vi "Digitizer Analyze_DCOffset.vi"(7 "Pins":string[](array[string])=["Xout"], 8 "error in (no error)":errorcluster, 9 "Published Data Id":string[](array[string]), 10 "Waveform Data In":waveform(dbl)[](array[waveform])=[{"t0"=timestamp(3637030365.2340937 s since 1904-01-01), "dt"=3.3333333333333334e-08, "Y"=array[5343 elements]}, {"t0"=timestamp(3637030365.2340937 s since 1904-01-01), "dt"=3.3333333333333334e-08, "Y"=array[5343 elements]}], 11 "Semiconductor Module Context":T1) -> (0 "error out":errorcluster, 3 "DCOffset":dbl[](array[numeric]))   [LabVIEW 2014]
doc: "Example: Measurement Library\n\nRecommended Input Signal: 100 kHz, 2 Vpp, sine wave\n\nDevices Supported: Refer to NI Example Finders\n\nLabVIEW Description:\n\nThis example illustrates fetching scalar measurements from NI-SCOPE, such as period and rise time calculations. \n\nSome common horizontal and vertical parameters are configured for the oscilloscope. The property node is used to set the reference level units, and the low, middle and high reference levels. For more information about measurement library parameters, see the NI-SCOPE VI Reference Help file. \n\nAfter the Read VI is called to acquire a waveform, the Fetch Measurement Stats VI is used to perform the desired scalar measurement analysis on the waveform. NI-SCOPE keeps a history of each measurement's results, which allows it to retrieve the statistics computed over multiple acquisitions. These statistics include the mean, standard deviation, min, max and number of acquisitions used in the statistics. The statistics are updated once per acquisition when the measurement is fetched. The Clear Stats VI clears this history."
uses:
  <vilib>/NI_TestStand_SemiconductorModule/NI_TestStand_Semiconductor_Module.lvlibp/PinMap/General/SemiconductorModuleContext.ctl
  <vilib>/NI_TestStand_SemiconductorModule/NI_TestStand_Semiconductor_Module.lvlibp/PinMap/General/NIInstrumentTypeIDs.ctl
  <vilib>/measure/madcrms.llb/Basic Averaged DC-RMS for 1 Chan.vi
  <vilib>/NI_TestStand_SemiconductorModule/NI_TestStand_Semiconductor_Module.lvlibp/PinMap/General/Publish/PublishDataDoubleFunctionalTest.vi
  <vilib>/NI_TestStand_SemiconductorModule/NI_TestStand_Semiconductor_Module.lvlibp
  <vilib>/measure/NI_MAPro.lvlib
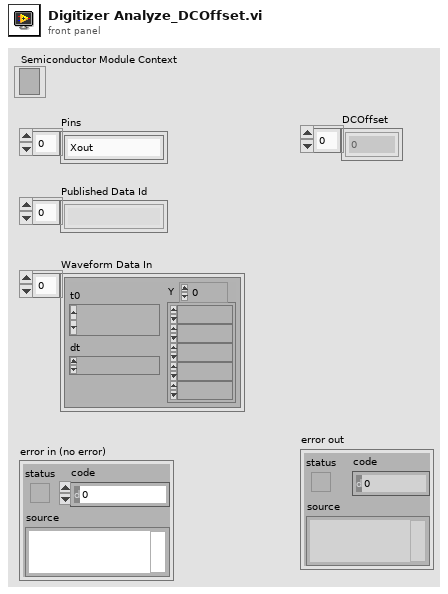
[diagram p1: front panel]
types:
  T1 = typedef "NI_TestStand_Semiconductor_Module.lvlibp/SemiconductorModuleContext.ctl" = refnum<k7>
  T2 = typedef "NI_TestStand_Semiconductor_Module.lvlibp/NIInstrumentTypeIDs.ctl" = string
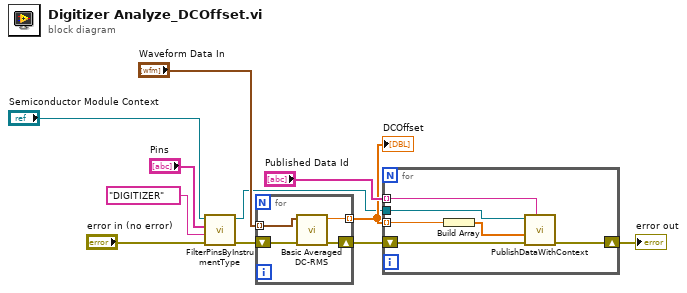
[diagram p0: block diagram]
diagram:
  n1 = call <vilib>:"FilterPinsByInstrumentType.vi"("error in (no error)"="error in (no error)", "Instrument Type Id"=T2 "DIGITIZER", "Pins"="Pins", "Semiconductor Module Context"="Semiconductor Module Context") -> ("error out"=w4:errorcluster, "Semiconductor Module Context Out"=w2:T1)  [unwired: 5 in, 1 out]
  n2 = for {
    tunnel: "Waveform Data In" -> [w15] mode=indexing
    tunnel: [w14] -> w5 mode=indexing
    shift-right: [w12] -> w3
    shift-left: w4 -> [w13]
    n3 = call-poly <vilib>:"Basic Averaged DC-RMS.vi"("error in (no error)"=w13, "signal in"=w15) -> ("error out"=w12:errorcluster, "DC value"=w14:dbl)  [unwired: 6 in, 2 out]
  }
  "DCOffset" <- w5
  n4 = for {
    tunnel: "Published Data Id" -> [w21] mode=indexing
    shift-right: [w19] -> w7
    shift-left: w3 -> [w20]
    tunnel: w5 -> [w17] mode=indexing
    tunnel: w2 -> [w16]
    n5 = Build Array(w17) -> (w18:dbl[])
    n6 = call-poly <vilib>:"PublishDataWithContext.vi"("Published Data Id"=w21, "error in (no error)"=w20, "Data In"=w18, "Semiconductor Module Context"=w16) -> ("error out"=w19:errorcluster)  [unwired: 6 in, 1 out]
  }
  "error out" <- w7
